vi "Init Config.vi"(8 "error in":errorcluster) -> (0 "error out":errorcluster, 3 "Configuration":T1)   [LabVIEW 2020, in "Acquisition.lvlib" / "Configuration.lvclass"]
doc: "Initialize the configuration for this module.\n____\nPeloton Config 2.0.0.9\nCopyright (c) 2024, Peloton"
uses:
  Configuration.lvclass
  Configuration--cluster.ctl
  C:/Program Files (x86)/National Instruments/LabVIEW 2020/vi.lib/Peloton/Peloton Config/DCFG Framework/Configuration_class/Configuration.lvclass
  <vilib>/Peloton/Peloton Config/DCFG Framework/Configuration_class/Configuration.lvclass/Configuration.ctl
  Configuration.lvclass/Configuration.ctl
  <vilib>/Peloton/Peloton Config/DCFG Framework/Configuration_class/Set Name.vi
  <vilib>/Peloton/Peloton Config/DCFG Framework/Configuration_class/Set File.vi
  <vilib>/Peloton/Peloton Config/DCFG Framework/Configuration_class/Set Order.vi
  <vilib>/Peloton/Peloton Config/DCFG Framework/Configuration_class/Set UIs.vi
  <vilib>/Peloton/Peloton Config/DCFG Framework/Configuration_class/Set Views.vi
  Set Configuration.vi
  UI - Configuration.vi
  UI - Settings.vi
  <vilib>/Peloton/Peloton Config/DCFG Framework/Peloton_lib_DCFG Framework.lvlib
  <vilib>/Peloton/Peloton Config/DCFG Framework/Configuration_class/Configuration.lvclass
  Acquisition.lvlib
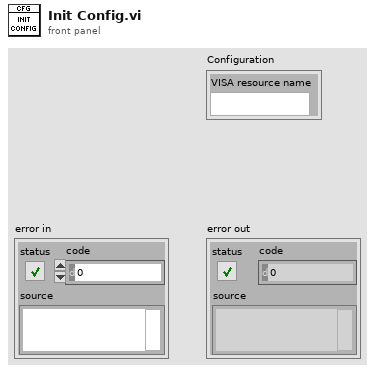
[diagram p1: front panel]
types:
  T1 = typedef "Acquisition.lvlib/Configuration.lvclass/Configuration--cluster.ctl" = cluster{"VISA resource name":refnum<visa-resource-name>}
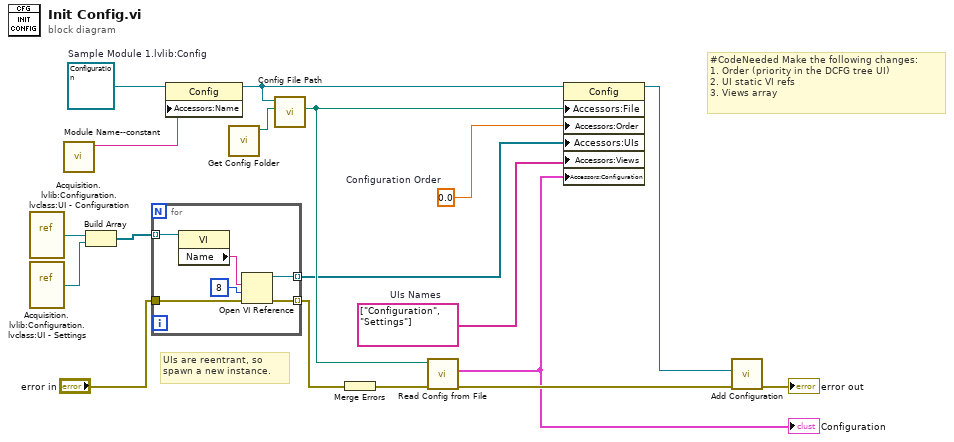
[diagram p0: block diagram]
diagram:
  w15 = string[] ["Configuration", "Settings"]  # UIs Names
  w17 = 0.0  # Configuration Order
  w14 = refnum<class "Configuration.lvclass"> refnum  # Sample Module 1.lvlib:Config
  # "UIs are reentrant, so spawn a new instance."
  # "#CodeNeeded Make the following changes:\n1. Order (priority in the DCFG tree UI)\n2. UI static VI refs\n3. Views array"
  n1 = vi-ref "Acquisition.lvlib:Configuration.lvclass:UI - Configuration.vi"() -> (w2:refnum<vi>)
  n2 = vi-ref "Acquisition.lvlib:Configuration.lvclass:UI - Settings.vi"() -> (w1:refnum<vi>)
  n3 = call "Module Name--constant.vi"() -> ("Module Name"=w9:string)  [unwired: 11 in]
  n4 = Build Array "Build Array"(w2, w1) -> (w7:refnum<vi>[])
  n5 = for {
    tunnel: [w22] -> w4 mode=indexing
    tunnel: w7 -> [w19] mode=indexing
    tunnel: "error in" -> [w24]
    tunnel: [w23] -> w5 mode=indexing
    n6 = property class="VI"(reference=w19) -> ("Name"=w20:string)  [unwired: 1 in, 2 out]
    n7 = Open VI Reference(vi path=w20, options=8, error in (no error)=w24) -> (vi reference=w22:refnum<vi>, error out=w23:errorcluster)  [unwired: 3 in]
  }
  n8 = property class="Config"(reference=w14, "Accessors:Name"=w9) -> (reference out=w10:refnum<class "Configuration.lvclass">)  [unwired: 1 in, 1 out]
  n9 = call <vilib>:"Get Config Folder.vi"() -> ("Config Folder"=w3:path)  [unwired: 9 in, 2 out]
  n10 = call <vilib>:"Config File Path.vi"("Config Folder"=w3, "Config"=w10) -> ("Config File Path"=w16:path)  [unwired: 9 in]
  n11 = Merge Errors(w5) -> (w8:errorcluster)
  n12 = call "Read Config from File.vi"("error in"=w8, "Config File"=w16) -> ("error out"=w12:errorcluster, "Configuration"=w11:T1)  [unwired: 8 in]
  "Configuration" <- w11
  n13 = property class="Config"(reference=w10, "Accessors:File"=w16, "Accessors:Order"=w17, "Accessors:UIs"=w4, "Accessors:Views"=w15, "Accessors:Configuration"=w11) -> (reference out=w13:refnum<class "Configuration.lvclass">)  [unwired: 1 in, 1 out]
  n14 = call <vilib>:"Add Configuration.vi"("error in"=w12, "Config"=w13) -> ("error out"=→"error out":errorcluster)  [unwired: 9 in]
